vi "Lvlib Save for Previous.vi"(7 "Target Version":string="15.0", 8 "Error In":errorcluster, 10 "Destination Folder":path, 11 "Original lvlib":path) -> (0 "Error Out":errorcluster)   [LabVIEW 2017]
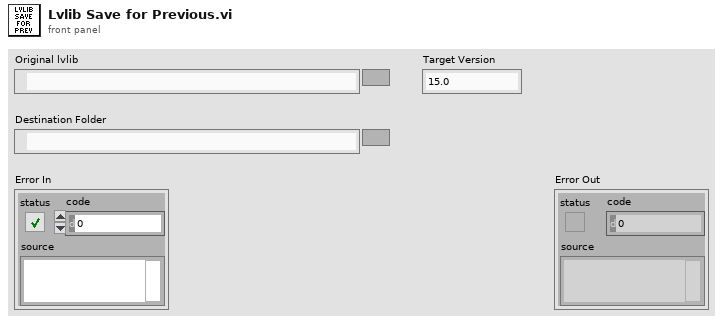
[diagram p1: front panel]
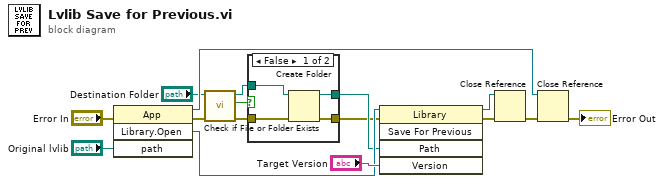
[diagram p0: block diagram]
diagram:
  n1 = invoke class="App" method="Library.Open"(error in="Error In", "path"="Original lvlib") -> (reference out=w12:refnum<vi>, error out=w7:errorcluster, "Open Library"=w14:refnum<vi>)  [unwired: 2 in, 1 out]
  n2 = call <vilib>:"Check if File or Folder Exists.vi"("error in (no error)"=w7, "path"="Destination Folder") -> ("error out"=w2:errorcluster, "file or folder exists?"=w6:bool, "dup path"=w5:path)  [unwired: 7 in]
  n3 = case shown="False" w6 {
    tunnel: w5 -> [w20 w22]
    tunnel: [w19 w22] -> w3
    tunnel: w2 -> [w18 w21]
    tunnel: [w17 w21] -> w1
    frame False {
      n4 = Create Folder(path (use dialog)=w20, error in=w18) -> (created path=w19:path, error out=w17:errorcluster)  [unwired: 1 in, 1 out]
    }
    frame True {
    }
  }
  n5 = invoke class="Library" method="Save For Previous"(reference=w14, error in=w1, "Path"=w3, "Version"="Target Version") -> (reference out=w10:refnum<vi>, error out=w11:errorcluster)  [unwired: 1 in, 3 out]
  n6 = Close Reference(reference=w10, error in (no error)=w11) -> (error out=w13:errorcluster)
  n7 = Close Reference(reference=w12, error in (no error)=w13) -> (error out=→"Error Out":errorcluster)
